vi "Main Action Que_NmeArr.vi"(7 "Action":enum16{"Initial", "Add", "Release"}(ring)=enum."Release", 8 "error in (no error)":errorcluster, 11 "Process":string[](array[string])) -> (0 "error out":errorcluster, 3 "Process Que Out":refnum<queue>)   [LabVIEW 2019]
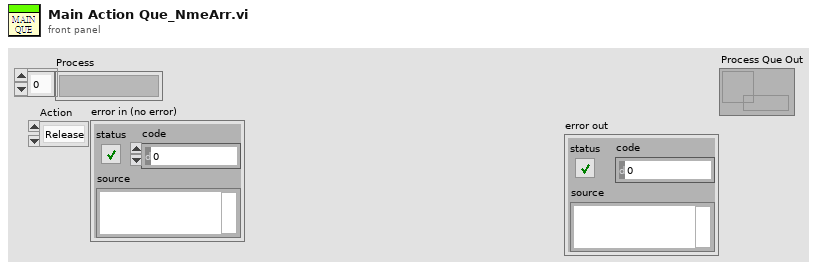
[diagram p1: front panel]
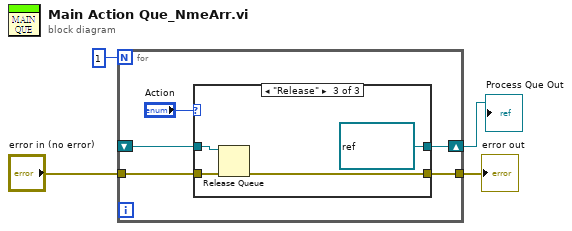
[diagram p0: block diagram]
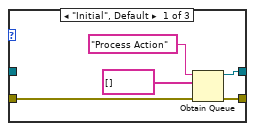
[diagram p2: hidden frame]
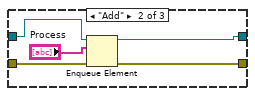
[diagram p3: hidden frame]
diagram:
  n1 = for {
    N: 1 -> [_]
    shift-right: [w9] -> w3
    shift-left: _ -> [w8]
    tunnel: "error in (no error)" -> [w6]
    tunnel: [w5] -> w1
    n2 = case shown="\"Release\"" "Action" {
      tunnel: [w12 w18 refnum<queue> refnum ("queue out")] -> w9
      tunnel: w8 -> [_ w19 w23]
      tunnel: w6 -> [w11 w15 w21]
      tunnel: [w10 w16 w22] -> w5
      frame "Initial", Default {
        n3 = Obtain Queue(name (unnamed)="Process Action", element data type=string[] [], error in (no error)=w11) -> (queue out=w12:refnum<queue>, error out=w10:errorcluster)  [unwired: 2 in, 1 out]
      }
      frame "Add" {
        n4 = Enqueue Element(queue=w19, element="Process", error in (no error)=w15) -> (queue out=w18:refnum<queue>, error out=w16:errorcluster)  [unwired: 1 in, 1 out]
      }
      frame "Release" {
        n5 = Release Queue(queue=w23, error in (no error)=w21) -> (error out=w22:errorcluster)  [unwired: 1 in, 2 out]
      }
    }
  }
  "error out" <- w1
  "Process Que Out" <- w3
